vi "Send Header to Self.vi"(8 "error in":errorcluster, 10 "Header":string, 11 "File Actor in":refnum<class "File Actor.lvclass">) -> (0 "error out":errorcluster, 3 "File Actor out":refnum<class "File Actor.lvclass">)   [LabVIEW 2017, in "File Library.lvlib" / "File Actor.lvclass"]
doc: "Wrapper for sending a message to self to write the header data."
uses:
  File Actor.lvclass
  C:/Program Files (x86)/National Instruments/LabVIEW 2017/vi.lib/ActorFramework/Actor/Actor.lvclass
  Messages/To/Update File Header MSG/Update Header MSG.lvclass
  C:/Program Files (x86)/National Instruments/LabVIEW 2017/vi.lib/ActorFramework/Message/Message.lvclass
  Messages/To/Update File Header MSG/Update Header MSG.lvclass/Update Header MSG.ctl
  <vilib>/ActorFramework/Actor/Actor.lvclass/Actor.ctl
  <vilib>/ActorFramework/Message Enqueuer/Message Enqueuer.lvclass/Message Enqueuer.ctl
  Messages/To/Update File Header MSG/Write Header.vi
  <vilib>/ActorFramework/Message Enqueuer/Init from Existing Queue.vi
  <vilib>/ActorFramework/Message Priority Queue/Priority Enqueue.vi
  <vilib>/ActorFramework/Message Enqueuer/Message Enqueuer.lvclass
  <vilib>/ActorFramework/Actor/Actor.lvclass
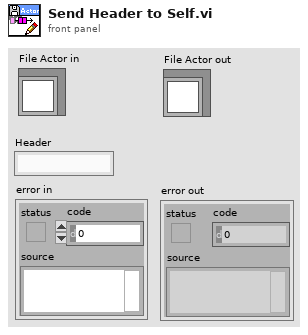
[diagram p1: front panel]
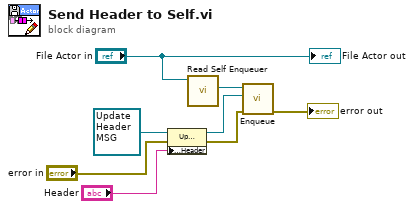
[diagram p0: block diagram]
diagram:
  n1 = property class="Update Header"(reference=refnum<class "Update Header MSG.lvclass"> refnum ("File Library.lvlib:Update Header"), error in="error in", "Accessors:Header"="Header") -> (reference out=w4:refnum<class "Update Header MSG.lvclass">, error out=w1:errorcluster)
  n2 = call <vilib>:"Read Self Enqueuer.vi"("Actor"="File Actor in") -> ("Self Enqueuer"=w7:refnum<class "Message Enqueuer.lvclass">)  [unwired: 10 in]
  n3 = call <vilib>:"Enqueue.vi"("error in (no error)"=w1, "Message"=w4, "Message Enqueuer in"=w7) -> ("error out"=→"error out":errorcluster)  [unwired: 7 in, 1 out]
  "File Actor out" <- "File Actor in"
